vi "uC_support.vi"() -> ()   [LabVIEW 2012]
uses:
  meas_date.vi
panel:
  in  "Tab Control":T1(tab)
  in  "exit":bool
  out "Wynonywanie pomiarów":bool
  out "Zebranych pomiarów":u64
  out "Połączenie bluetooth":bool
  in  "Bt button":bool
  in  "Measurment button":bool
  in  "Terminate the program":bool
  out "voltage":cluster{"No.":u64, "Voltage":dbl}[](graph)
  out "temperature":T2(graph)
  out "current":cluster{"No.":u64, "Current":dbl}[](graph)
  out "Temperature 2":dbl
  out "Temperature":dbl
  out "Voltage":dbl
  out "Current":dbl
  out "Current":dbl(knob) scale=0.0..8.0
  out "Voltage":dbl(knob) scale=0.0..20.0
  out "Thermometer":dbl(slide) scale=0.0..100.0
  out "Thermometer 2":dbl(slide) scale=0.0..100.0
  in  "'<' or '>'":enum16{"less than", "greater than"}(ring)
  in  "ending condition sets":T3(tab)
  in  "amount":u32=1000
  in  "temperature 1":dbl
  in  "temperature 2":dbl
  in  "voltage":dbl
  in  "current":dbl
  in  "type":T3(ring)
  out "meter reading\nfrequancy":dbl
  in  "meter reading\nfrequancy":dbl(knob)=0.1 min=0.1 max=1000000.0 scale=0.1..1000000.0
  in  "refresh bt wait ms":u32=1
  in  "check ms delay for start measurment":u32=1
  in  "id pin":T4(ring)=enum."ADC7"
  in  "id pin":T4(ring)=enum."ADC6"
  in  "id pin":T4(ring)=enum."ADC5"
  in  "voltage \nreferences":enum16{"2,56", "5,00"}(ring)
  in  "measurment delay ms":u32=1000
  in  "commands details":T5(array[cluster])=[{"id"=0, "name"="status", "params"=[], "respons char"=["command id", "DDRA", "DDRB", "DDRC", "DDRD", "PORTA", "PORTB", "PORTC", "PORTD"]}, {"id"=1, "name"="voltometer", "params"=[{"name"="ADC pin", "count"=3}, {"name"="vol ref", "count"=1}], "respons char"=["command id", "low result", "high result"]}, {"id"=2, "name"="temperature", "params"=[{"name"="ADC pin", "count"=3}, {"name"="id pin", "count"=3}], "respons char"=["command id", "low result", "high result"]}]
  out "close error":errorcluster
  out "open error":errorcluster
  out "reapons char error":errorcluster
  out "check buffer error":errorcluster
  out "sending error":errorcluster
  out "reapons char error 2":errorcluster
  out "check buffer error 2":errorcluster
  out "sending error 2":errorcluster
  out "sending error 3":errorcluster
  out "check buffer error 3":errorcluster
  out "reapons char error 3":errorcluster
  # "Przytrzymaj by przerwać"
  # "temperature 1"
  # "temperature 2"
  # "voltage"
  # "current"
  # "voltage"
  # "bluetooth"
  # "temperature 1"
  # "temperature 2"
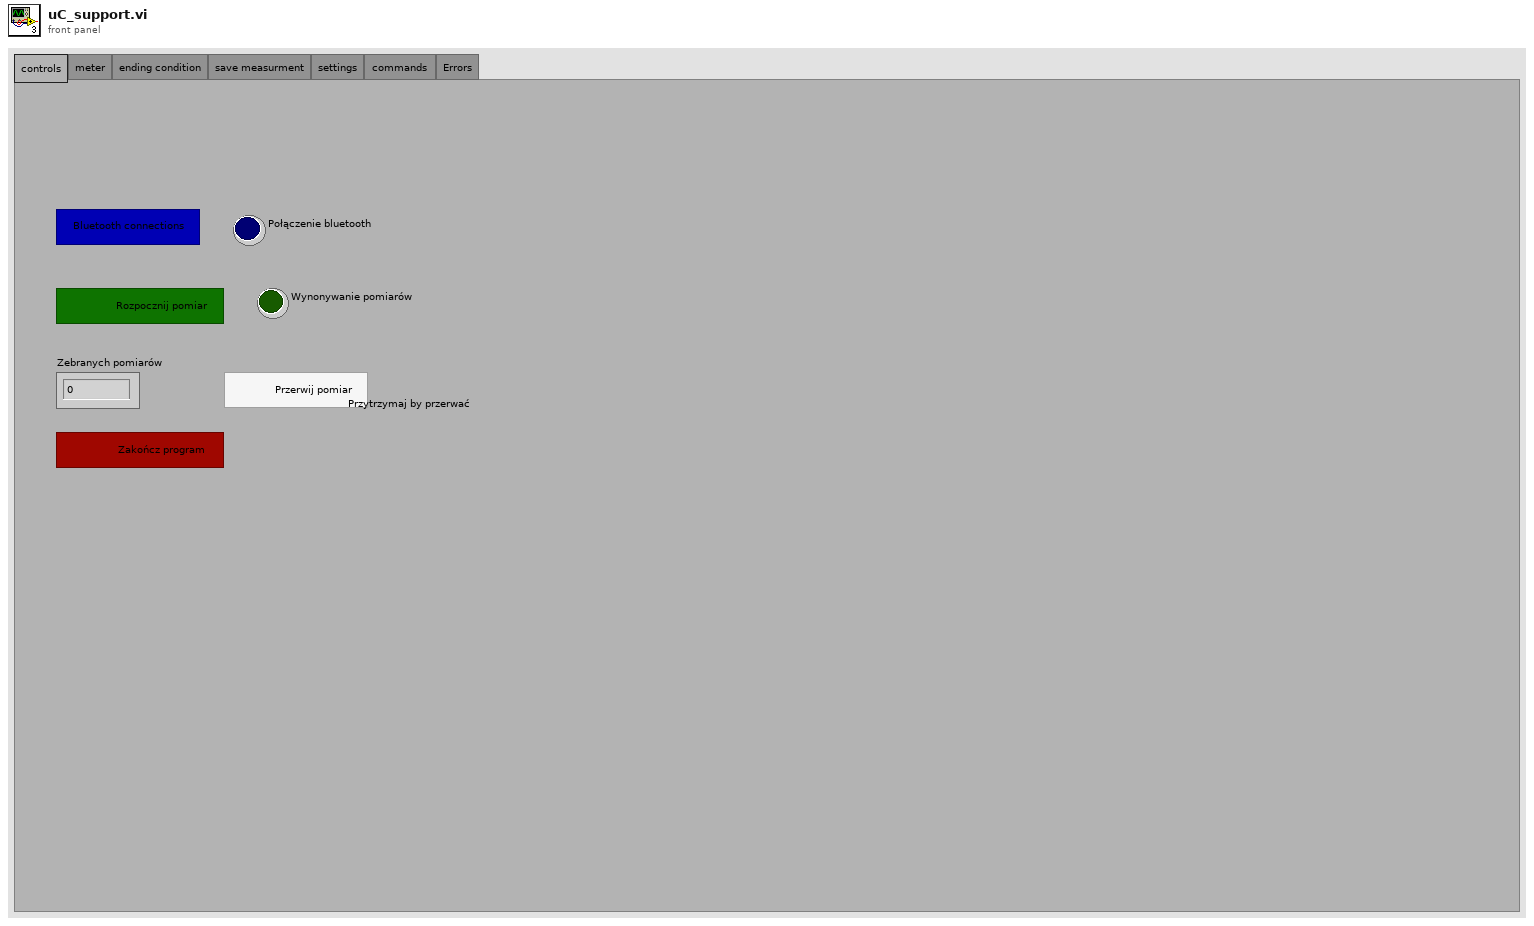
[diagram p1: front panel]
types:
  T1 = enum32{"controls", "meter", "ending condition", "save measurment", "settings", "commands ", "Errors"}
  T2 = cluster{"No.":u64, "Temperature":dbl, "Temperature 2":dbl}[]
  T3 = enum32{"amount", "time", "temperature 1", "temperature 2", "voltage", "current"}
  T4 = enum16{"ADC0", "ADC1", "ADC2", "ADC3", "ADC4", "ADC5", "ADC6", "ADC7"}
  T5 = cluster{"id":u8, "name":string, "params":cluster{"name":string, "count":u8}[], "respons char":string[]}[]
  T6 = cluster{"No.":u64, "Voltage":dbl, "Current":dbl, "time":dbl, "Temperature":dbl, "Temperature 2":dbl}
  T7 = cluster{"No.":u64, "Temperature":dbl, "Temperature 2":dbl}
  T8 = cluster{"No.":u64, "Voltage":dbl, "Current":dbl, "time":dbl, "Temperature":dbl, "Temperature 2":dbl}[]
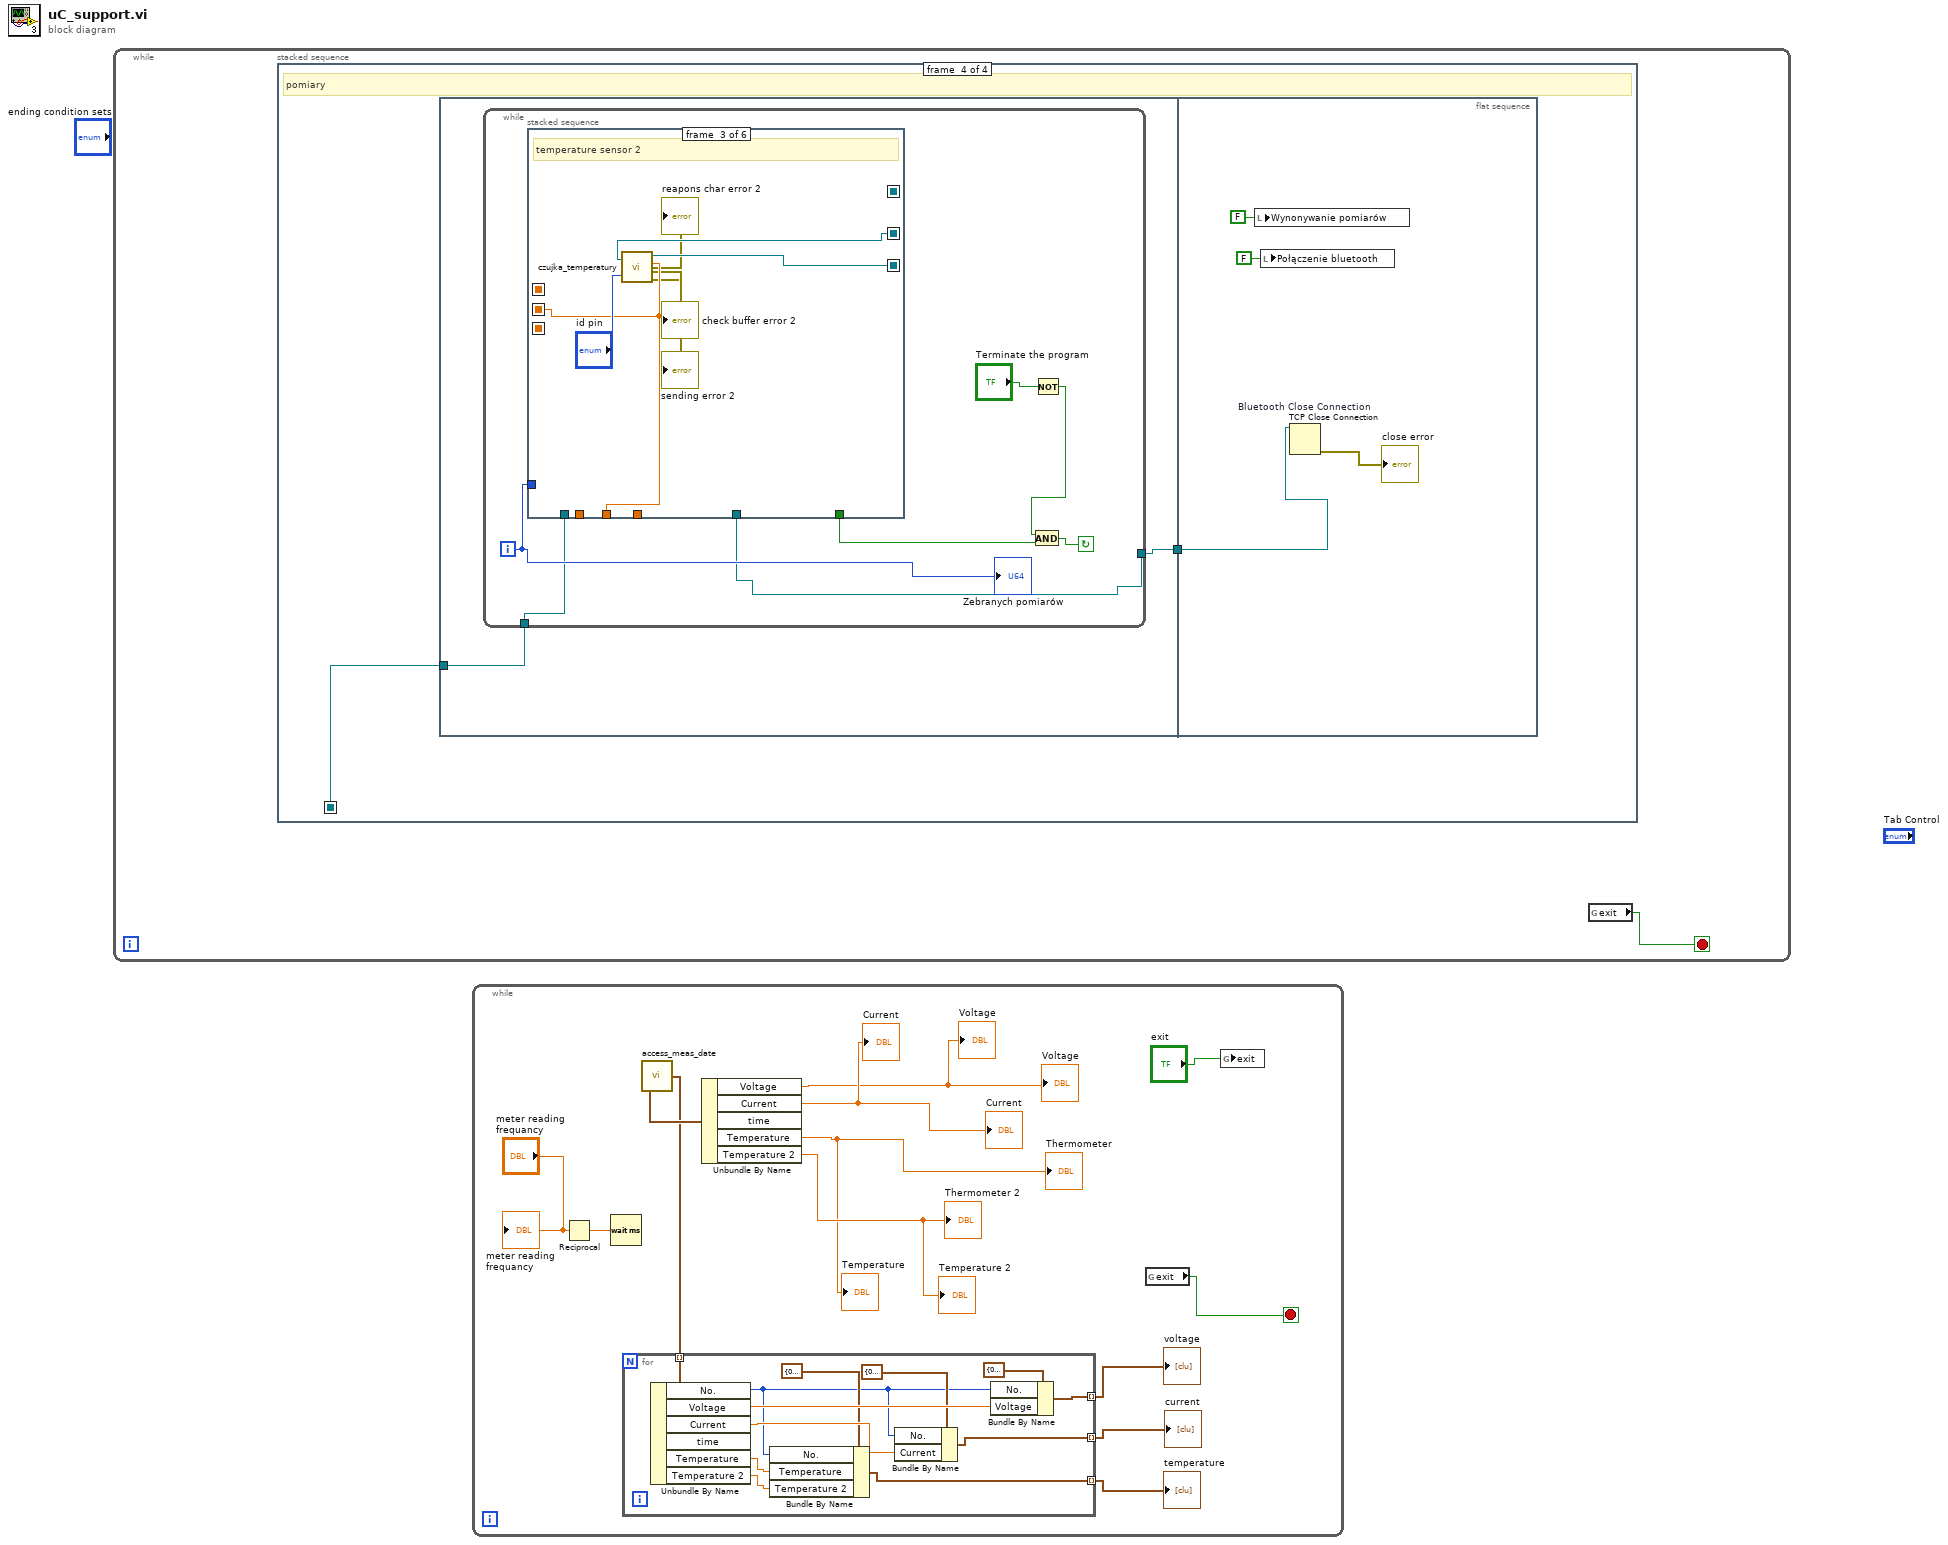
[diagram p0: block diagram]
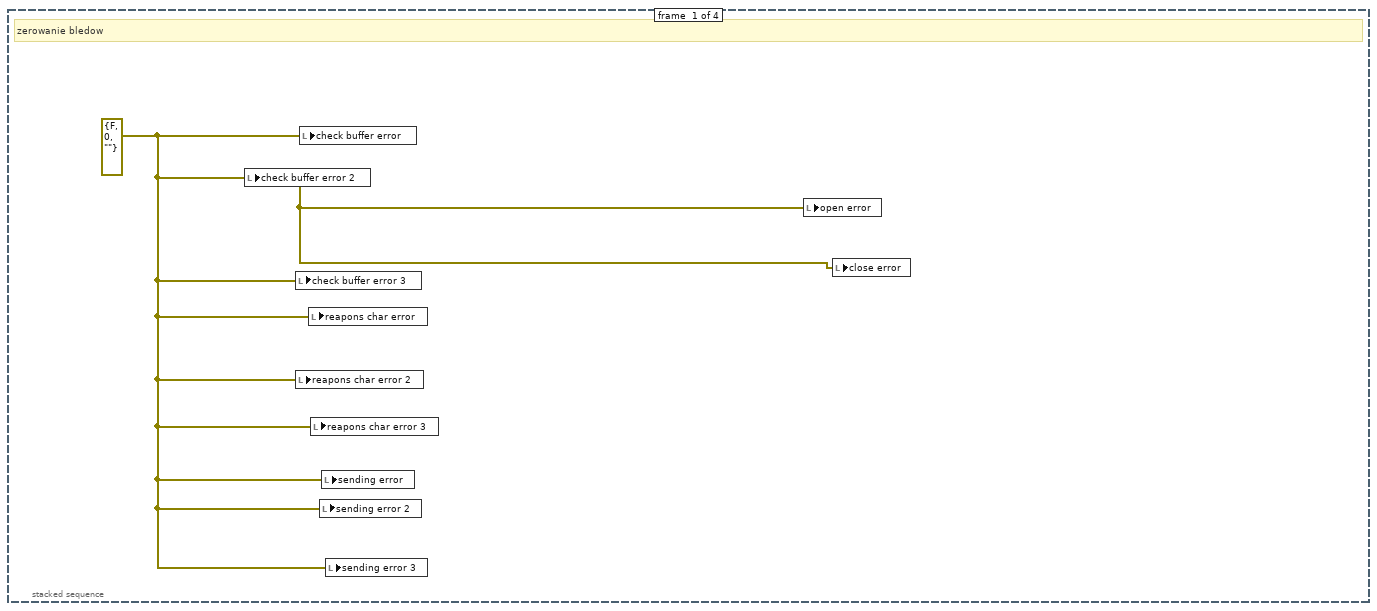
[diagram p2: hidden frame]
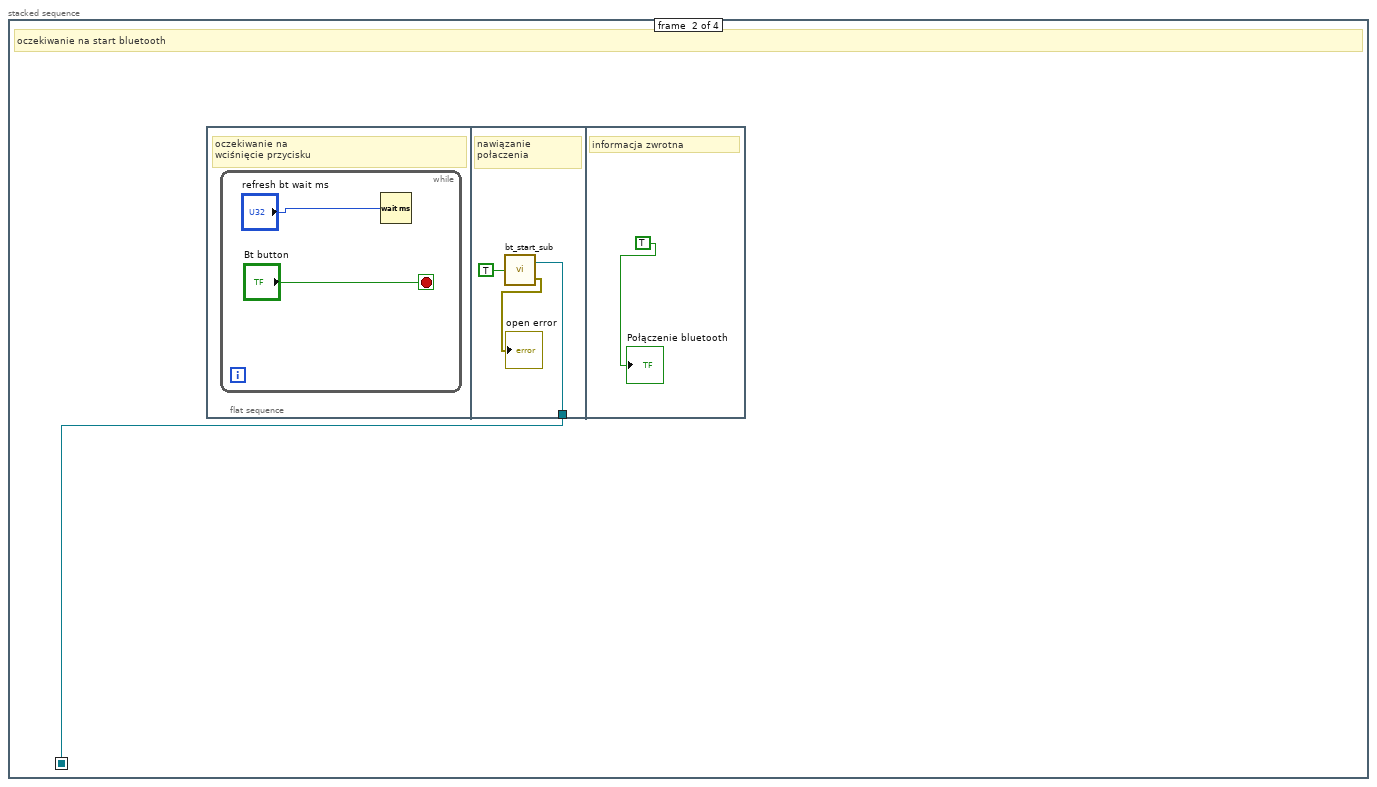
[diagram p3: hidden frame]
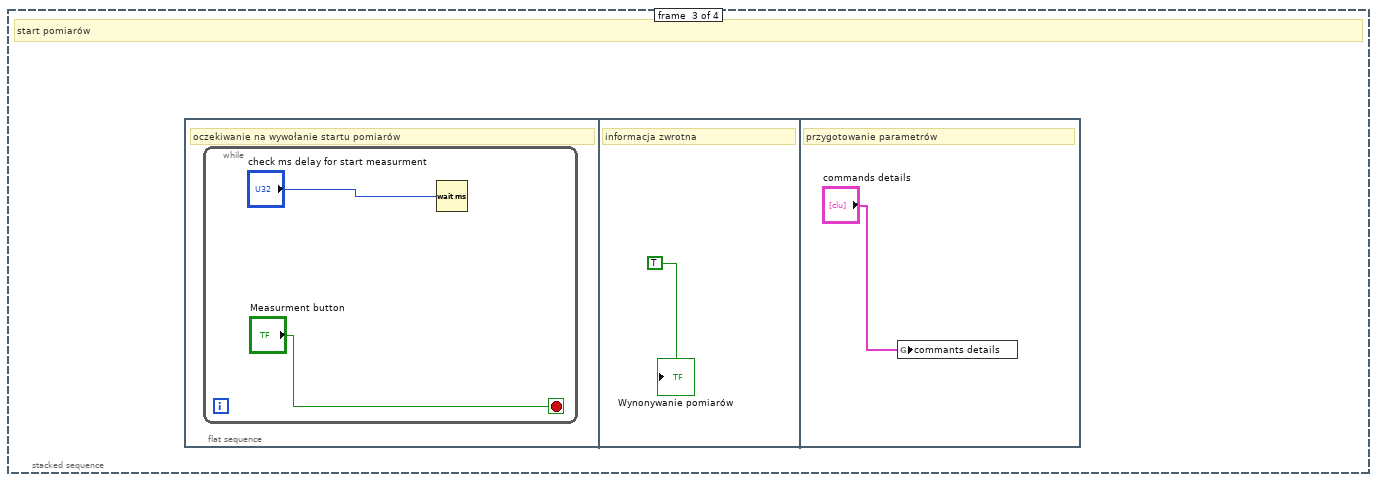
[diagram p4: hidden frame]
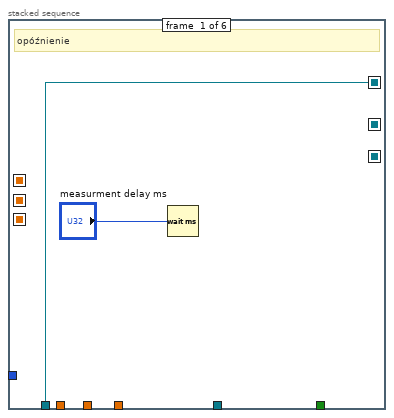
[diagram p5: hidden frame]
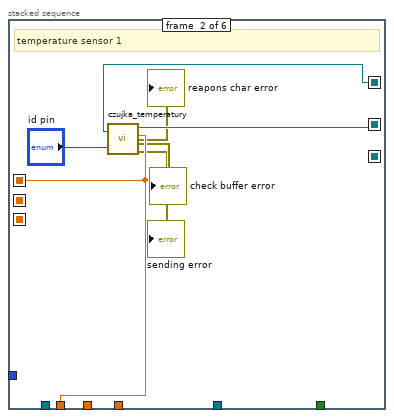
[diagram p6: hidden frame]
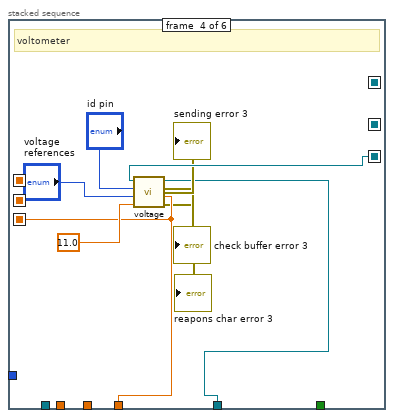
[diagram p7: hidden frame]
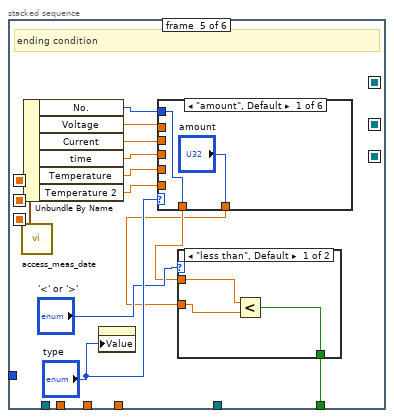
[diagram p8: hidden frame]
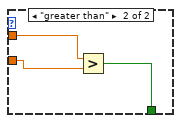
[diagram p9: hidden frame]
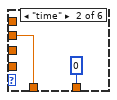
[diagram p10: hidden frame]
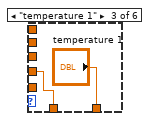
[diagram p11: hidden frame]
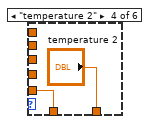
[diagram p12: hidden frame]
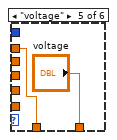
[diagram p13: hidden frame]
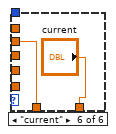
[diagram p14: hidden frame]
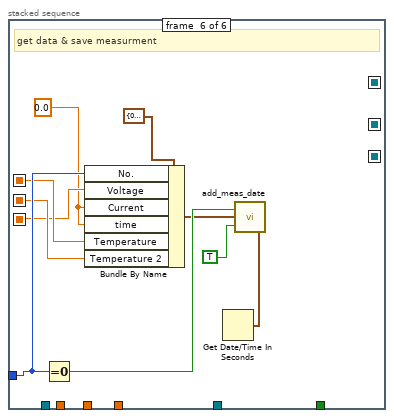
[diagram p15: hidden frame]
diagram:
  n1 = while {
    stop <- w1 stop-if-true
    n2 = stacked-sequence {
      seq-local: [_ w3 _ _] -> [_ _ _ w14]
      frame #0 {
        w2 = errorcluster {"status"=FALSE, "code"=0, "source"=""} ("check buffer error")
        # "zerowanie bledow"
        n3 = local write "check buffer error 2"(w2) -> ()
        n4 = local write "check buffer error 3"(w2) -> ()
        n5 = local write "reapons char error 2"(w2) -> ()
        n6 = local write "check buffer error"(w2) -> ()
        n7 = local write "reapons char error"(w2) -> ()
        n8 = local write "reapons char error 3"(w2) -> ()
        n9 = local write "sending error 2"(w2) -> ()
        n10 = local write "sending error"(w2) -> ()
        n11 = local write "sending error 3"(w2) -> ()
        n12 = local write "open error"(w2) -> ()
        n13 = local write "close error"(w2) -> ()
      }
      frame #1 {
        # "oczekiwanie na start bluetooth"
        n14 = flat-sequence {
          tunnel: [w6] -> w3
          frame #0 {
            # "oczekiwanie na \nwciśnięcie przycisku"
            n15 = while {
              stop <- "Bt button" stop-if-true
              n16 = Wait (ms)(milliseconds to wait="refresh bt wait ms") -> ()  [unwired: 1 out]
            }
          }
          frame #1 {
            # "nawiązanie połaczenia"
            n17 = call "bt_start_sub.vi"("auto?"=TRUE) -> ("connection ID"=w6:refnum<k31>, "open error"=→"open error":errorcluster)
          }
          frame #2 {
            # "informacja zwrotna"
            "Połączenie bluetooth" <- TRUE
          }
        }
      }
      frame #2 {
        # "start pomiarów"
        n18 = flat-sequence {
          frame #0 {
            # "oczekiwanie na wywołanie startu pomiarów"
            n19 = while {
              stop <- "Measurment button" stop-if-true
              n20 = Wait (ms)(milliseconds to wait="check ms delay for start measurment") -> ()  [unwired: 1 out]
            }
          }
          frame #1 {
            # "informacja zwrotna"
            "Wynonywanie pomiarów" <- TRUE
          }
          frame #2 {
            # "przygotowanie parametrów"
            n21 = global write "meas_date.vi" "commants details"("commands details") -> ()
          }
        }
      }
      frame #3 {
        # "pomiary"
        n22 = flat-sequence {
          tunnel: w14 -> [w17]
          tunnel: [w16] -> w15
          tunnel: w15 -> [w90]
          frame #0 {
            n23 = while {
              tunnel: w17 -> [w20]
              tunnel: [w19] -> w16
              i -> [w21]
              stop <- w22 continue-if-true
              n24 = stacked-sequence {
                seq-local: [_ _ w39 _ _ _] -> [_ _ _ w49 _ _]
                seq-local: [_ w33 _ _ _ _] -> [_ _ w40 _ _ _]
                seq-local: [_ w31 _ _ _ _] -> [_ _ _ _ _ w83]
                seq-local: [_ _ w37 _ _ _] -> [_ _ _ _ _ w82]
                seq-local: [_ _ _ w45 _ _] -> [_ _ _ _ _ w81]
                seq-local: [w25 _ _ _ _ _] -> [_ w27 _ _ _ _]
                tunnel: [_ w31 _ _ _ _] -> _
                tunnel: [_ _ w37 _ _ _] -> _
                tunnel: [_ _ _ w45 _ _] -> _
                tunnel: [_ _ _ w41 _ _] -> w19
                tunnel: [_ _ _ _ w50 _] -> w18
                tunnel: w21 -> [_ _ _ _ _ w84]
                tunnel: w20 -> [w25 _ _ _ _ _]
                frame #0 {
                  # "opóźnienie"
                  n25 = Wait (ms)(milliseconds to wait="measurment delay ms") -> ()  [unwired: 1 out]
                }
                frame #1 {
                  # "temperature sensor 1"
                  n26 = call "czujka_temperatury.vi"("id pin"="id pin", "connection in"=w27) -> ("sending error"=→"sending error":errorcluster, "check buffer error"=→"check buffer error":errorcluster, "temperature"=w31:dbl, "connection out"=w33:refnum<k31>, "reapons char error"=→"reapons char error":errorcluster)
                }
                frame #2 {
                  # "temperature sensor 2"
                  n27 = call "czujka_temperatury.vi"("id pin"="id pin", "connection in"=w40) -> ("sending error"=→"sending error 2":errorcluster, "check buffer error"=→"check buffer error 2":errorcluster, "temperature"=w37:dbl, "connection out"=w39:refnum<k31>, "reapons char error"=→"reapons char error 2":errorcluster)
                }
                frame #3 {
                  # "voltometer"
                  n28 = call "voltage.vi"("connection in"=w49, "id pin"="id pin", "voltage \nreferences"="voltage \nreferences", "divider"=11.0) -> ("sending error"=→"sending error 3":errorcluster, "connection out"=w41:refnum<k31>, "check buffer error"=→"check buffer error 3":errorcluster, "voltage"=w45:dbl, "reapons char error"=→"reapons char error 3":errorcluster)
                }
                frame #4 {
                  # "ending condition"
                  n29 = call "access_meas_date.vi"() -> ("last measurment"=w61:T6)  [unwired: 1 out]
                  n30 = Unbundle By Name(w61) -> ("No."=w60:u64, "Voltage"=w59:dbl, "Current"=w58:dbl, "time"=w54:dbl, "Temperature"=w57:dbl, "Temperature 2"=w56:dbl)
                  n31 = property class="Enum (strict)"("Value"="type") -> ()  [unwired: 2 in, 2 out]
                  n32 = case shown="\"amount\", Default" "type" {
                    tunnel: w60 -> [w69 _ _ _ _ _]
                    tunnel: w59 -> [_ _ _ _ w76 _]
                    tunnel: w58 -> [_ _ _ _ _ w78]
                    tunnel: w54 -> [_ w71 _ _ _ _]
                    tunnel: w57 -> [_ _ w72 _ _ _]
                    tunnel: w56 -> [_ _ _ w74 _ _]
                    tunnel: [w69 w71 w72 w74 w76 w78] -> w52
                    tunnel: ["amount" u32 0 ("amount") "temperature 1" "temperature 2" "voltage" "current"] -> w51
                    frame "amount", Default {
                    }
                    frame "time" {
                    }
                    frame "temperature 1" {
                    }
                    frame "temperature 2" {
                    }
                    frame "voltage" {
                    }
                    frame "current" {
                    }
                  }
                  n33 = case shown="\"less than\", Default" "'<' or '>'" {
                    tunnel: w51 -> [w63 w66]
                    tunnel: w52 -> [w64 w67]
                    tunnel: [w62 w65] -> w50
                    frame "less than", Default {
                      n34 = Less?(x=w64, y=w63) -> (x < y?=w62:bool)
                    }
                    frame "greater than" {
                      n35 = Greater?(x=w67, y=w66) -> (0:w65:bool)
                    }
                  }
                }
                frame #5 {
                  w80 = 0.0 ("time")
                  # "get data & save measurment"
                  n36 = Equal To 0?(x=w84) -> (x = 0?=w87:bool)
                  n37 = Bundle By Name(cluster=T6 {"No."=0, "Voltage"=0.0, "Current"=0.0, "time"=0.0, "Temperature"=0.0, "Temperature 2"=0.0} ("measurment to add"), "No."=w84, "Voltage"=w81, "Current"=w80, "time"=w80, "Temperature"=w83, "Temperature 2"=w82) -> (w86:T6)
                  n38 = Get Date/Time In Seconds() -> (seconds since 1Jan1904=w89:timestamp)
                  n39 = call "add_meas_date.vi"("Data"=w89, "measurment to add"=w86, "to date?"=TRUE, "new?"=w87) -> ()
                }
              }
              n40 = Not(x="Terminate the program") -> (.not. x?=w23:bool)
              n41 = And(x=w23, y=w18) -> (x .and. y?=w22:bool)
              "Zebranych pomiarów" <- w21
            }
          }
          frame #1 {
            n42 = local write "Wynonywanie pomiarów"(FALSE ("Wynonywanie pomiarów")) -> ()
            n43 = local write "Połączenie bluetooth"(FALSE ("Połączenie bluetooth")) -> ()
            n44 = TCP Close Connection "Bluetooth Close Connection"(connection ID=w90) -> (error out=→"close error":errorcluster)  [unwired: 2 in, 1 out]
          }
        }
      }
    }
    n45 = global read "meas_date.vi" "exit"() -> (w1:bool)
  }
  n46 = while {
    stop <- w98 stop-if-true
    n47 = Reciprocal(x="meter reading\nfrequancy") -> (1/x=w105:dbl)
    n48 = Wait (ms)(milliseconds to wait=w105) -> ()  [unwired: 1 out]
    n49 = call "access_meas_date.vi"() -> ("last measurment table"=w97:T8, "last measurment"=w106:T6)
    n50 = for {
      tunnel: w97 -> [w118] mode=indexing
      tunnel: [w115] -> w96 mode=indexing
      tunnel: [w112] -> w95 mode=indexing
      tunnel: [w107] -> w94 mode=indexing
      n51 = Unbundle By Name(w118) -> ("No."=w110:u64, "Voltage"=w116:dbl, "Current"=w113:dbl, "Temperature"=w109:dbl, "Temperature 2"=w108:dbl)  [unwired: 1 out]
      n52 = Bundle By Name(cluster=T7 {"No."=0, "Temperature"=0.0, "Temperature 2"=0.0}, "No."=w110, "Temperature"=w109, "Temperature 2"=w108) -> (w107:T7)
      n53 = Bundle By Name(cluster=cluster{"No.":u64, "Current":dbl} {"No."=0, "Current"=0.0}, "No."=w110, "Current"=w113) -> (w112:cluster{"No.":u64, "Current":dbl})
      n54 = Bundle By Name(cluster=cluster{"No.":u64, "Voltage":dbl} {"No."=0, "Voltage"=0.0}, "No."=w110, "Voltage"=w116) -> (w115:cluster{"No.":u64, "Voltage":dbl})
    }
    "current" <- w95
    "temperature" <- w94
    "voltage" <- w96
    n55 = Unbundle By Name(w106) -> ("Voltage"=→"Voltage" →"Voltage":dbl, "Current"=→"Current" →"Current":dbl, "Temperature"=→"Thermometer" →"Temperature":dbl, "Temperature 2"=→"Thermometer 2" →"Temperature 2":dbl)  [unwired: 1 out]
    n56 = global read "meas_date.vi" "exit"() -> (w98:bool)
    n57 = global write "meas_date.vi" "exit"("exit") -> ()
    "meter reading\nfrequancy" <- "meter reading\nfrequancy"
  }
